vi "dump.vi"(8 "error in (no error)":errorcluster, 10 "indent":T1, 11 "NoneType in":refnum<class "NoneType.lvclass">) -> (0 "error out":errorcluster, 2 "mlir":string, 3 "NoneType out":refnum<class "NoneType.lvclass">)   [LabVIEW 2020, in "mlir.lvlib" / "NoneType.lvclass"]
uses:
  NoneType.lvclass
  Node/indent.ctl
  mlir.lvlib
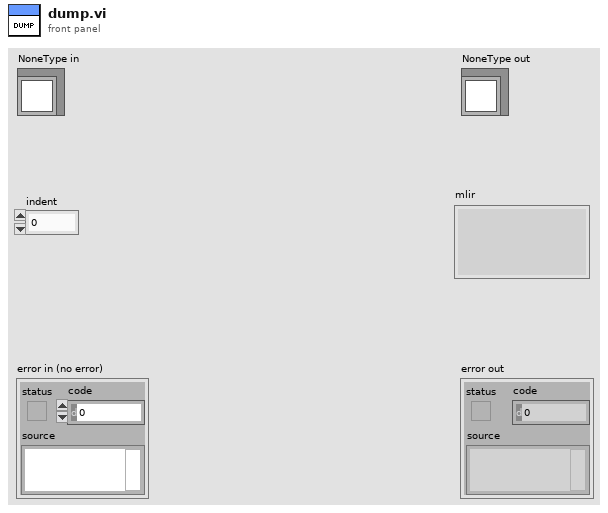
[diagram p1: front panel]
types:
  T1 = typedef "mlir.lvlib/indent.ctl" = u32
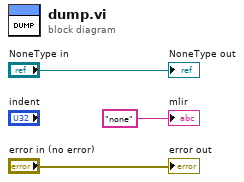
[diagram p0: block diagram]
diagram:
  "error out" <- "error in (no error)"
  "NoneType out" <- "NoneType in"
  "mlir" <- "none" ("mlir")
